vi "Write Sized Payload.vi"(8 "error in (no error)":errorcluster, 10 "Payload":string, 11 "TCP in":refnum<k5>) -> (0 "error out":errorcluster, 3 "TCP":refnum<k5>)   [LabVIEW 2020, in "Vecto.lvlib" / "TCPMessaging.lvclass"]
uses:
  TCPMessaging.lvclass
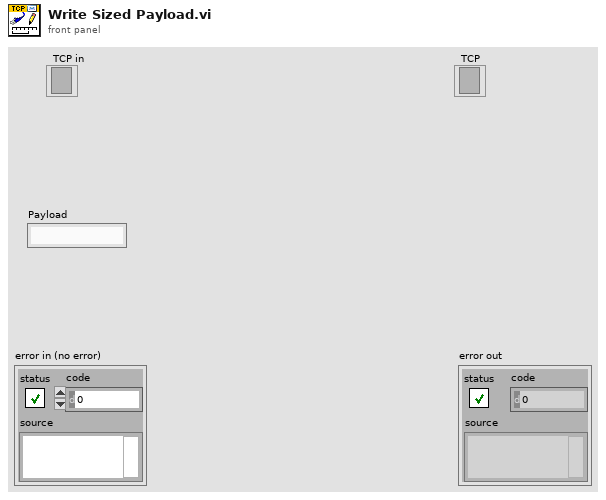
[diagram p1: front panel]
types:
  T1 = enum16{"big-endian, network order", "native, host order", "little-endian"}
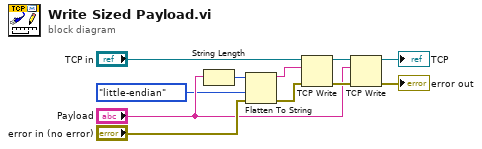
[diagram p0: block diagram]
diagram:
  n1 = String Length(string="Payload") -> (length=w10:i32)
  n2 = Flatten To String(anything=w10, byte order (0:big-endian, network order)=T1."little-endian", error in (no error)="error in (no error)") -> (data string=w9:string, error out=w3:errorcluster)  [unwired: 1 in, 1 out]
  n3 = TCP Write(connection ID="TCP in", data in=w9, error in (no error)=w3) -> (connection ID out=w8:refnum<k5>, error out=w7:errorcluster)  [unwired: 1 in, 1 out]
  n4 = TCP Write(connection ID=w8, data in="Payload", error in (no error)=w7) -> (connection ID out=→"TCP":refnum<k5>, error out=→"error out":errorcluster)  [unwired: 1 in, 1 out]
